vi "Time FGV(SubVI).vi"() -> ()   [LabVIEW 2017]
panel:
  in  "열거형":enum16{"초기화", "카운트", "정지"}(ring)
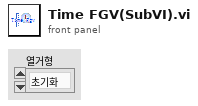
[diagram p1: front panel]
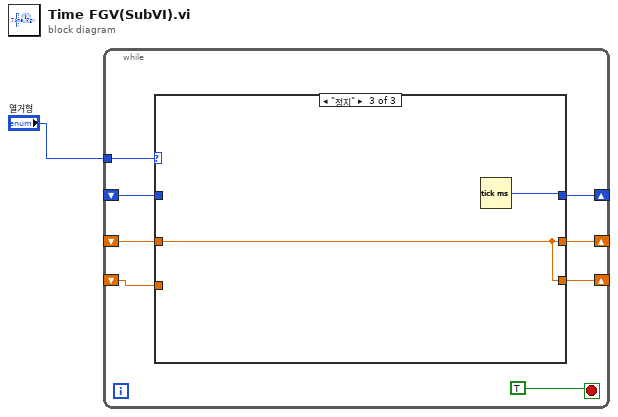
[diagram p0: block diagram]
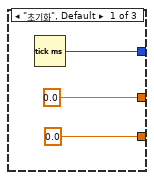
[diagram p2: hidden frame]
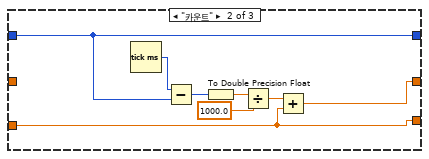
[diagram p3: hidden frame]
diagram:
  n1 = while {
    tunnel: "열거형" -> [w9]
    shift-right: [w8] -> _
    shift-left: _ -> [w5]
    shift-right: [w7] -> _
    shift-left: _ -> [w3]
    shift-right: [w6] -> _
    shift-left: _ -> [w4]
    stop <- TRUE stop-if-true
    n2 = case shown="\"정지\"" w9 {
      tunnel: [w12 w19 w22] -> w8
      tunnel: [0.0 w14 w21] -> w7
      tunnel: [0.0 w13 w21] -> w6
      tunnel: w5 -> [_ w19 _]
      tunnel: w4 -> [_ w13 _]
      tunnel: w3 -> [_ _ w21]
      frame "초기화", Default {
        n3 = Tick Count (ms)() -> (millisecond timer value=w12:u32)
      }
      frame "카운트" {
        n4 = Tick Count (ms)() -> (millisecond timer value=w20:u32)
        n5 = Subtract(x=w20, y=w19) -> (x-y=w18:u32)
        n6 = To Double Precision Float(number=w18) -> (double precision float=w17:dbl)
        n7 = Divide(x=w17, y=1000.0) -> (x/y=w15:dbl)
        n8 = Add(x=w15, y=w13) -> (x+y=w14:dbl)
      }
      frame "정지" {
        n9 = Tick Count (ms)() -> (millisecond timer value=w22:u32)
      }
    }
  }
